vi "Read string.vi"(7 "count (1)":i32, 8 "Error In":errorcluster, 9 "from (0:start)":enum16{"start", "end", "current"}(ring), 10 "offset (in bytes) (0)":i64, 11 "WFM file ref":T1={"refnum"=refnum, "byte order"=enum."little-endian", "Version"=0}) -> (0 "Error Out":errorcluster, 2 "data":string, 3 "WFM file ref out":T1={"refnum"=refnum, "byte order"=enum."little-endian", "Version"=0})   [LabVIEW 2015]
uses:
  WFM file ref.ctl
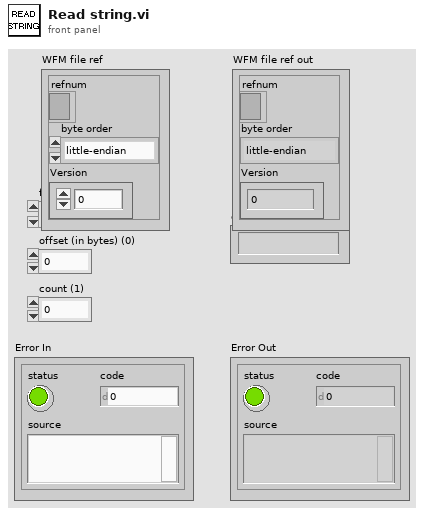
[diagram p1: front panel]
types:
  T1 = typedef "WFM file ref.ctl" = cluster{"refnum":refnum<file>, "byte order":enum16{"big-endian, network order", "native, host order", "little-endian"}, "Version":i32}
  T2 = enum16{"big-endian, network order", "native, host order", "little-endian"}
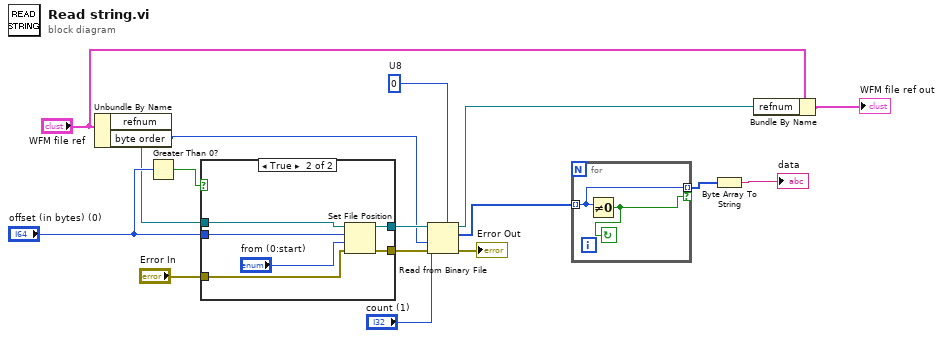
[diagram p0: block diagram]
diagram:
  w15 = u8 0  # U8
  n1 = Unbundle By Name("WFM file ref") -> ("refnum"=w5:refnum<file>, "byte order"=w4:T2)
  n2 = Greater Than 0?(x="offset (in bytes) (0)") -> (x > 0?=w11:bool)
  n3 = case shown="True" w11 {
    tunnel: w5 -> [w18 w24]
    tunnel: "offset (in bytes) (0)" -> [_ w23]
    tunnel: [w18 w21] -> w16
    tunnel: "Error In" -> [w17 w20]
    tunnel: [w17 w19] -> w13
    frame False {
    }
    frame True {
      n4 = Set File Position(offset (in bytes) (0)=w23, refnum=w24, from (0:start)="from (0:start)", error in=w20) -> (refnum out=w21:refnum<file>, error out=w19:errorcluster)
    }
  }
  n5 = Read from Binary File(5:w15, 8:w13, 9:w4, 10:"count (1)", 11:w16) -> (0:→"Error Out":errorcluster, 2:w8:u8[], 3:w2:refnum<file>)  [unwired: 1 in, 1 out]
  n6 = for {
    tunnel: w8 -> [w26] mode=indexing
    tunnel: [w26] -> w7 mode=indexing if=w25
    stop <- w25 continue-if-true
    n7 = Not Equal To 0?(x=w26) -> (x != 0?=w25:bool)
  }
  n8 = Byte Array To String(unsigned byte array=w7) -> (string=→"data":string)
  n9 = Bundle By Name(cluster="WFM file ref", "refnum"=w2) -> (→"WFM file ref out":T1)
